vi "Check-sample-rate.vi"(8 "error in":errorcluster, 10 "Config. params. ref.":refnum<data-value>, 11 "Acquis. params. ref.":refnum<data-value>) -> (0 "error IO":errorcluster, 3 "Passed?":bool)   [LabVIEW 2013, in "CameraVision.lvlib" / "CV-Acquisition.lvclass"]
uses:
  CV-Acquisition.lvclass
  Configuration/CV-Configuration.lvclass
  CV-Acquisition.lvclass/CV-Acquisition.ctl
  Configuration/CV-Configuration.lvclass/CV-Configuration.ctl
  Configuration/Read ROI height.vi
  Configuration/Read ROI width.vi
  Read Maximum frame rate.vi
  Read Trigger mode.vi
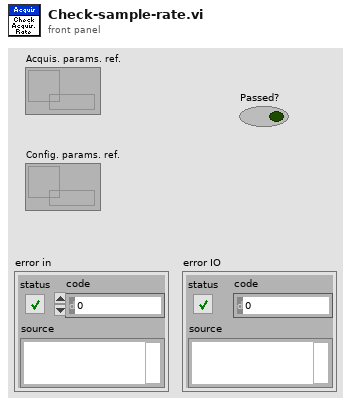
[diagram p1: front panel]
types:
  T1 = typedef "Trigger-modes.ctl" = enum16{"Camera timed (not sync.)", "Framegrabber timed (sync.)", "Software timed (sync.)", "External timing (sync.)", "Manual (sync.)", "Gated - camera (not sync.)", "Gated - grabber (sync.)", "Gated - software (sync.)", "Gated - external (sync.)"}
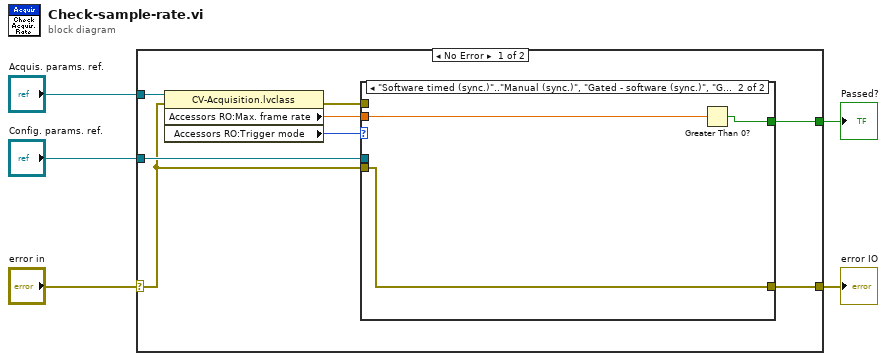
[diagram p0: block diagram]
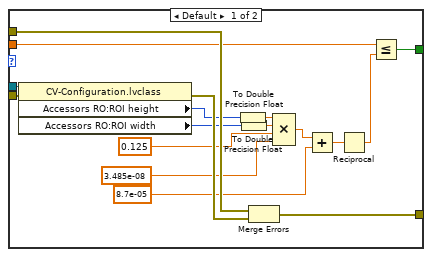
[diagram p2: hidden frame]
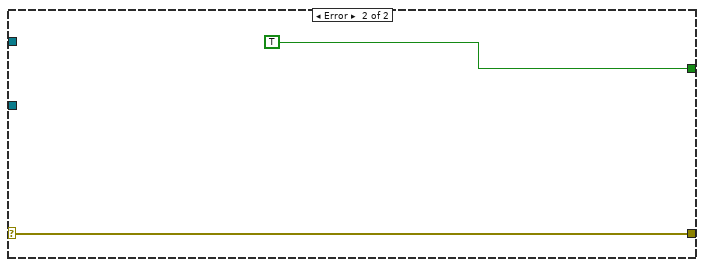
[diagram p3: hidden frame]
diagram:
  n1 = case shown="No Error" "error in" {
    selector: "error in" -> [w9 w35]
    tunnel: [w10 w35] -> w5
    tunnel: "Acquis. params. ref." -> [w13 _]
    tunnel: "Config. params. ref." -> [w12 _]
    tunnel: [w7 TRUE] -> w2
    frame No Error {
      n2 = property class="CV-Acquisition.lvclass"(reference=w13, error in=w9) -> (error out=w11:errorcluster, "Accessors RO:Max. frame rate"=w8:dbl, "Accessors RO:Trigger mode"=w6:T1)  [unwired: 1 out]
      n3 = case shown="\"Software timed (sync.)\"..\"Manual (sync.)\", \"Gated - software (sync.)\", \"Gated - external (sync.)\"" w6 {
        tunnel: w12 -> [w30 _]
        tunnel: w11 -> [w29 _]
        tunnel: [w27 w31] -> w10
        tunnel: w9 -> [w26 w31]
        tunnel: w8 -> [w15 w32]
        tunnel: [w14 w33] -> w7
        frame Default {
          n4 = property class="CV-Configuration.lvclass"(reference=w30, error in=w26) -> (error out=w28:errorcluster, "Accessors RO:ROI height"=w25:u32, "Accessors RO:ROI width"=w24:u32)  [unwired: 1 out]
          n5 = To Double Precision Float(number=w25) -> (double precision float=w22:dbl)
          n6 = To Double Precision Float(number=w24) -> (double precision float=w21:dbl)
          n7 = Merge Errors(w29, w28) -> (w27:errorcluster)
          n8 = Compound Arithmetic op=MULTIPLY(w22, w21, 0.125 ("value"), 3.485e-08 ("value")) -> (w19:dbl)
          n9 = Add(x=w19, y=8.7e-05) -> (x+y=w17:dbl)
          n10 = Reciprocal(x=w17) -> (1/x=w16:dbl)
          n11 = Less Or Equal?(x=w15, y=w16) -> (x <= y?=w14:bool)
        }
        frame "Software timed (sync.)".."Manual (sync.)", "Gated - software (sync.)", "Gated - external (sync.)" {
          n12 = Greater Than 0?(x=w32) -> (x > 0?=w33:bool)
        }
      }
    }
    frame Error {
    }
  }
  "Passed?" <- w2
  "error IO" <- w5
